vi "toggles.vi"(11 "Joystick Boolean":bool) -> (0 "Toggled Boolean":bool)   [LabVIEW 2014]
panel:
  in  "Timer":dbl
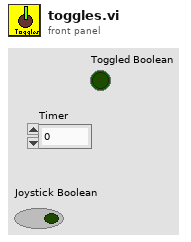
[diagram p1: front panel]
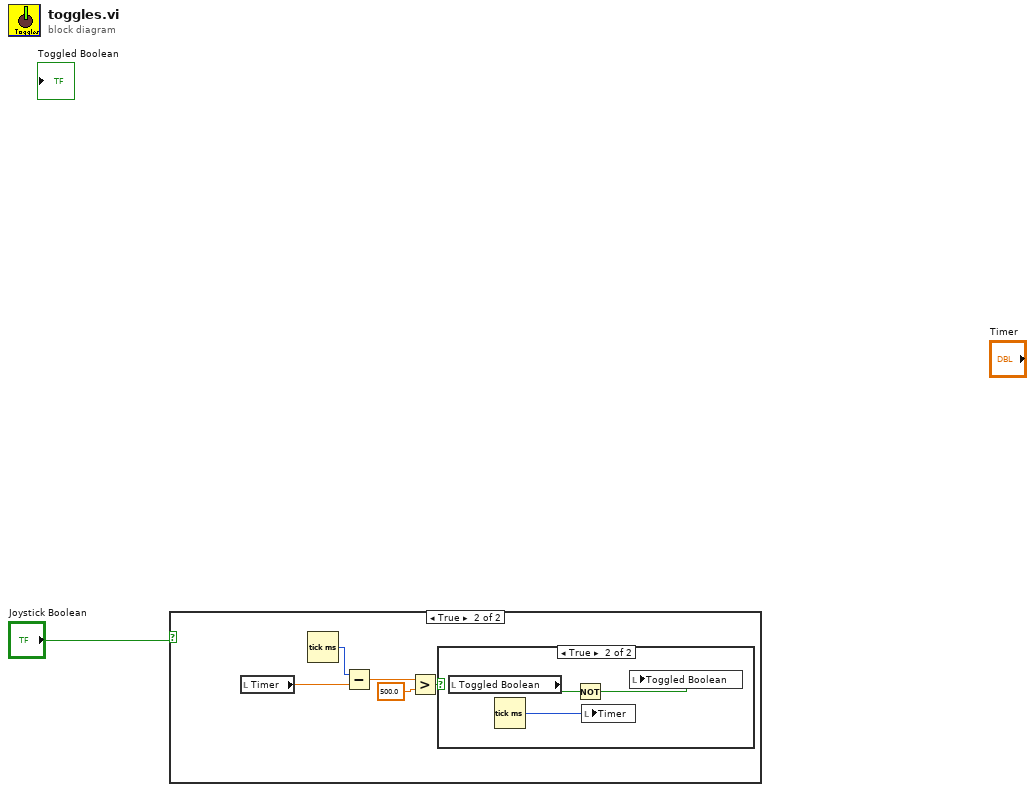
[diagram p0: block diagram]
diagram:
  n1 = case shown="True" "Joystick Boolean" {
    frame False {
    }
    frame True {
      n2 = local read "Timer"() -> (w5:dbl)
      n3 = Tick Count (ms)() -> (millisecond timer value=w6:u32)
      n4 = Subtract(x=w6, y=w5) -> (x-y=w4:dbl)
      n5 = Greater?(x=w4, y=500.0) -> (0:w2:bool)
      n6 = case shown="True" w2 {
        frame False {
        }
        frame True {
          n7 = local read "Toggled Boolean"() -> (w8:bool)
          n8 = Tick Count (ms)() -> (millisecond timer value=w9:u32)
          n9 = Not(x=w8) -> (.not. x?=w7:bool)
          n10 = local write "Timer"(w9) -> ()
          n11 = local write "Toggled Boolean"(w7) -> ()
        }
      }
    }
  }
